vi "Camera acquisition.vi"(0 "camera feed":T1, 5 "Stop (F)":bool, 7 "error in":errorcluster) -> (20 "Image Out":T2(plugin-control), 21 "All Image Buffers Out":refnum<image>[](array[refnum]), 22 "Image Number":u32, 25 "Frame Rate":dbl, 26 "Stopped":bool, 27 "error out":errorcluster)   [LabVIEW 2010]
doc: "Creates, and edits acquisitions using the NI Vision Acquisition Express VI.\n\nThe NI Vision Acquisition Wizard is launched by placing the Express VI on the block diagram. Select an acquisition source and configure an acquisition using NI-IMAQ, NI-IMAQdx, or simulate an acquisition by reading an AVI or image files from a folder. After an acquisition is configured, select controls and indicators to be able to programmatically set in LabVIEW. Double-click the Vision Acquisition Express VI to edit the acquisition.\n\nNote: Any images created by the Express VI need to be disposed after use. Use the IMAQ Dispose.vi to cleanup the images output by the Express VI when they are no longer needed."
uses:
  <vilib>/userDefined/High Color/IMAQdx.ctl
  <vilib>/vision/driver/NI_Vision_Acquisition_Software.lvlib
  Program Files (x86)/National Instruments/LabVIEW 2010/resource/objmgr/imaqdx.rc
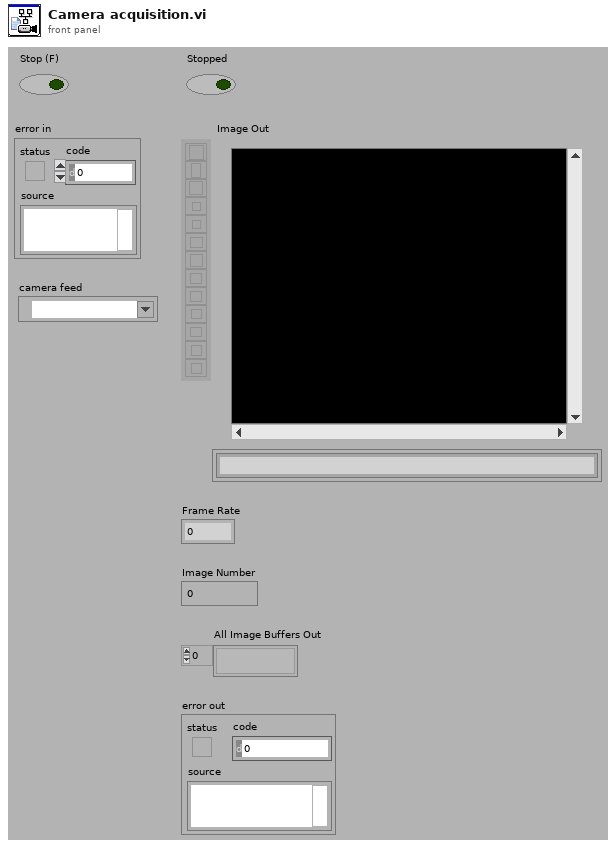
[diagram p1: front panel]
types:
  T1 = typedef "IMAQdx.ctl" = refnum<k21>
  T2 = typedef "IMAQ Image.ctl" = refnum<image>
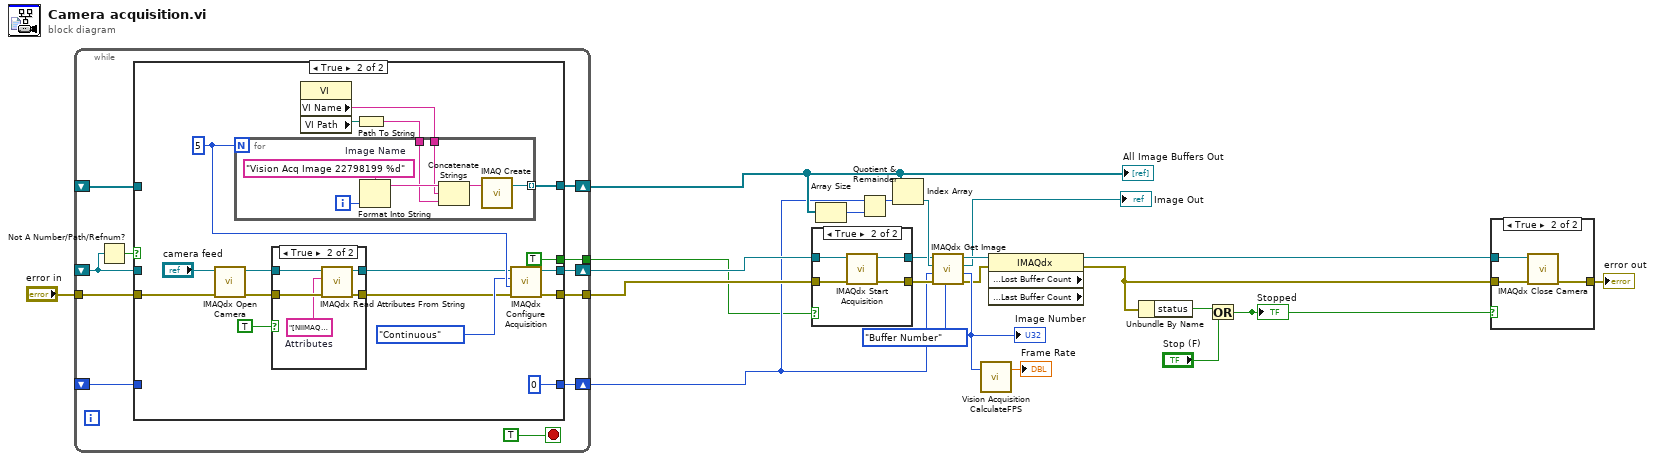
[diagram p0: block diagram]
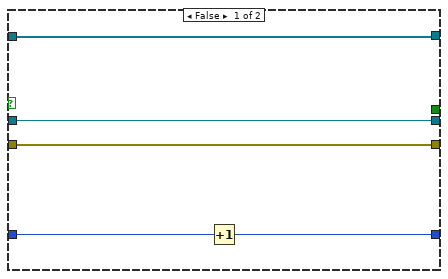
[diagram p4: hidden frame]
diagram:
  n1 = while {
    shift-right: [w34] -> w8
    shift-left: _ -> [w26]
    tunnel: [w33] -> w22
    tunnel: "error in" -> [w32]
    shift-right: [w30] -> w12
    shift-left: _ -> [w29]
    shift-right: [w28] -> w5
    shift-left: _ -> [w27]
    tunnel: [w24] -> w4
    stop <- TRUE stop-if-true
    n2 = Not A Number/Path/Refnum?(number/path/refnum=w26) -> (NaN/Path/Refnum?=w25:bool)
    n3 = case shown="True" w25 {
      tunnel: [w39 w55] -> w34
      tunnel: w26 -> [w39 _]
      tunnel: [w38 w54] -> w33
      tunnel: w32 -> [w38 w56]
      tunnel: [w37 w53] -> w30
      tunnel: w29 -> [w37 _]
      tunnel: [w35 0] -> w28
      tunnel: w27 -> [w36 _]
      tunnel: [_ TRUE] -> w24
      frame False {
        n4 = Increment(x=w36) -> (x+1=w35:i32)
      }
      frame True {
        w52 = u32 5 ("Number of Image Buffers")
        n5 = call <vilib>:"IMAQdx Open Camera.vi"("error in"=w56, "Session In"="camera feed") -> ("error out"=w45:errorcluster, "Session Out"=w46:T1)  [unwired: 1 in, 7 out]
        n6 = case shown="True" TRUE ("Init Attributes") {
          tunnel: w46 -> [w58 w63]
          tunnel: w45 -> [w57 w62]
          tunnel: [w58 w60] -> w44
          tunnel: [w57 w59] -> w43
          frame False {
          }
          frame True {
            w61 = "[NIIMAQ_HEADER]\nType = 2\nVersion = 8\n\n[CAMERA_DATA]\nAcquisitionAttributes::Bayer::GainB = \"1\"\nAcquisitionAttributes::Bayer::GainG = \"1\"\nAcquisitionAttributes::Bayer::GainR = \"1\"\nAcquisitionAttributes::Bayer::Pattern = \"Use hardware value\"\nAcquisitionAttributes::BitsPerPixel = \"Use hardware value\"\nAcquisitionAttributes::IgnoreFirstFrame = \"false\"\nAcquisitionAttributes::OverwriteMode = \"Get Newest\"\nAcquisitionAttributes::PixelSignedness = \"Signed\"\nAcquisitionAttributes::ReceiveTimestampMode = \"None\"\nAcquisitionAttributes::ShiftPixelBits = \"false\"\nAcquisitionAttributes::SwapPixelBytes = \"false\"\nAcquisitionAttributes::Timeout = \"5000\"\nAcquisitionAttributes::VerticalMirror = \"false\"\nAcquisitionAttributes::VideoMode = \"1280x800 YUY2 10.00fps\"\nCameraAttributes::BacklightCompensation::Mode = \"Manual\"\nCameraAttributes::BacklightCompensation::Value = \"false\"\nCameraAttributes::Brightness::Mode = \"Manual\"\nCameraAttributes::Brightness::Value = \"133\"\nCameraAttributes::Contrast::Mode = \"Manual\"\nCameraAttributes::Contrast::Value = \"0.050000000000000003\"\nCameraAttributes::Exposure::Mode = \"Auto\"\nCameraAttributes::Focus::Mode = \"Auto\"\nCameraAttributes::Pan::Mode = \"Manual\"\nCameraAttributes::Pan::Value = \"0\"\nCameraAttributes::Saturation::Mode = \"Manual\"\nCameraAttributes::Saturation::Value = \"83\"\nCameraAttributes::Sharpness::Mode = \"Manual\"\nCameraAttributes::Sharpness::Value = \"20\"\nCameraAttributes::Tilt::Mode = \"Manual\"\nCameraAttributes::Tilt::Value = \"0\"\nCameraAttributes::WhiteBalance::Mode = \"Auto\"\nCameraAttributes::Zoom::Mode = \"Manual\"\nCameraAttributes::Zoom::Value = \"0\"\n"  # Attributes
            n7 = call <vilib>:"IMAQdx Read Attributes From String.vi"("error in"=w62, "Attributes String In"=w61, "Session In"=w63) -> ("error out"=w59:errorcluster, "Session Out"=w60:T1)  [unwired: 7 out]
          }
        }
        n8 = property class="VI"() -> ("VI Name"=w48:string, "VI Path"=w49:path)  [unwired: 2 in, 2 out]
        n9 = Path To String(path=w49) -> (string=w47:string)
        n10 = for "For Loop_template0" {
          N: w52 -> [_]
          tunnel: [w70] -> w53 mode=indexing
          tunnel: w48 -> [w65]
          tunnel: w47 -> [w64]
          i -> [w69]
          w68 = "Vision Acq Image 22798199 %d"  # Image Name
          n11 = Format Into String(format string=w68, w69) -> (resulting string=w67:string)  [unwired: 2 in, 1 out]
          n12 = Concatenate Strings(w67, w65, w64) -> (w66:string)
          n13 = call "IMAQ Create"("Image Name"=w66) -> ("New Image"=w70:T2)  [unwired: 3 in, 2 out]
        }
        n14 = call <vilib>:"IMAQdx Configure Acquisition.vi"("error in"=w43, "Number of Buffers"=w52, "Continuous?"=enum32{"One Shot", "Continuous"}."Continuous" ("Mode"), "Session In"=w44) -> ("error out"=w54:errorcluster, "Session Out"=w55:T1)  [unwired: 6 out]
      }
    }
  }
  "All Image Buffers Out" <- w12
  n15 = case shown="True" w4 {
    tunnel: w8 -> [w72 w76]
    tunnel: w22 -> [w71 w75]
    tunnel: [w71 w74] -> w6
    tunnel: [w72 w73] -> w7
    frame False {
    }
    frame True {
      n16 = call <vilib>:"IMAQdx Start Acquisition.vi"("error in"=w75, "Session In"=w76) -> ("error out"=w74:errorcluster, "Session Out"=w73:T1)  [unwired: 8 out]
    }
  }
  n17 = Array Size(array=w12) -> (size(s)=w13:i32)
  n18 = Quotient & Remainder(x=w5, y=w13) -> (x-y*floor(x/y)=w11:i32)  [unwired: 1 out]
  n19 = Index Array(array=w12, index=w11) -> (element=w10:T2)
  n20 = call <vilib>:"IMAQdx Get Image.vi"("Buffer Number Mode (Next)"=enum32{"Next", "Last", "Buffer Number"}."Buffer Number" ("Buffer Number Mode (Next)_template1"), "error in"=w6, "Buffer Number In"=w5, "Image In"=w10, "Session In"=w7) -> ("error out"=w15:errorcluster, "Buffer Number Out"=w19:u32, "Image Out"=→"Image Out":T2, "Session Out"=w16:T1)  [unwired: 3 out]
  "Image Number" <- w19
  n21 = call <vilib>:"Vision Acquisition CalculateFPS.vi"("buffer number"=w19) -> ("acquired FPS"=→"Frame Rate":dbl)  [unwired: 2 out]
  n22 = property class="IMAQdx" props=["Status Information:Lost Buffer Count", "Status Information:Last Buffer Count"](reference=w16, error in=w15) -> (reference out=w3:T1, error out=w9:errorcluster)  [unwired: 2 out]
  n23 = Unbundle By Name(w9) -> ("status"=w21:bool)
  n24 = Or(x=w21, y="Stop (F)") -> (x .or. y?=w2:bool)
  "Stopped" <- w2
  n25 = case "Case Structure_template1" shown="True" w2 {
    tunnel: [w77 w79] -> w1
    tunnel: w9 -> [w77 w80]
    tunnel: w3 -> [_ w78]
    frame False {
    }
    frame True {
      n26 = call <vilib>:"IMAQdx Close Camera.vi"("error in"=w80, "Session In"=w78) -> ("error out"=w79:errorcluster)  [unwired: 9 out]
    }
  }
  "error out" <- w1
